vi "RM.serverInitialize.vi"(8 "error in":errorcluster, 11 "Item Ref in":T1 format="%.0x") -> (0 "error out":errorcluster, 3 "Item Ref out":T1 format="%.0x")   [LabVIEW 2016, in "FPGA Resource Manager.lvlib"]
uses:
  FPGA Resource Manager.lvlib
  <vilib>/NI Veristand/Custom Device API/Custom Device Item Ref.ctl
  RM.Globals.vi
  <vilib>/NI Veristand/Custom Device API/Set Item Property (String).vi
  <vilib>/NI Veristand/Custom Device API/Custom Device API.lvlib
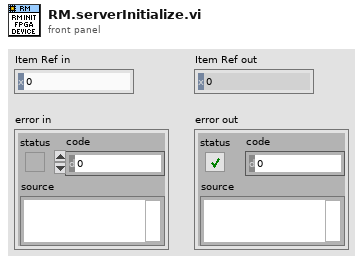
[diagram p1: front panel]
types:
  T1 = typedef "Custom Device API.lvlib/Custom Device Item Ref.ctl" = u64
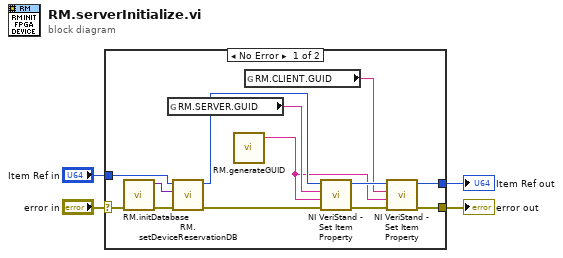
[diagram p0: block diagram]
diagram:
  n1 = case shown="No Error" "error in" {
    selector: "error in" -> [w15 w18]
    tunnel: "Item Ref in" -> [w17 w19]
    tunnel: [w7 w19] -> w3
    tunnel: [w9 w18] -> w1
    frame No Error {
      n2 = call "RM.initDatabase.vi"("error in"=w15) -> ("error out"=w16:errorcluster, "reservation DB out"=w13:variant)  [unwired: 9 in]
      n3 = global read "RM.Globals.vi" "RM.SERVER.GUID"() -> (w11:string)
      n4 = call "RM.setDeviceReservationDB.vi"("error in"=w16, "reservation DB in"=w13, "Item Ref in"=w17) -> ("error out"=w14:errorcluster, "Item Ref out"=w12:T1)  [unwired: 6 in, 1 out]
      n5 = call "RM.generateGUID.vi"() -> ("GUID"=w5:string)  [unwired: 2 in]
      n6 = global read "RM.Globals.vi" "RM.CLIENT.GUID"() -> (w6:string)
      n7 = call-poly <vilib>:"NI VeriStand - Set Item Property.vi"("error in (no error)"=w14, "Value"=w5, "Property Name"=w11, "Item Ref in"=w12) -> ("error out"=w10:errorcluster, "Item Ref out"=w8:T1)  [unwired: 5 in, 1 out]
      n8 = call-poly <vilib>:"NI VeriStand - Set Item Property.vi"("error in (no error)"=w10, "Value"=w5, "Property Name"=w6, "Item Ref in"=w8) -> ("error out"=w9:errorcluster, "Item Ref out"=w7:T1)  [unwired: 5 in, 1 out]
    }
    frame Error {
    }
  }
  "error out" <- w1
  "Item Ref out" <- w3
